vi "detect.vi"(0 "LS1":bool, 1 "Start":bool, 5 "LS2":bool, 7 "LS3":bool, 9 "LS4":bool, 11 "LS5":bool, 12 "Stop":bool) -> (6 "輸出":T1)   [LabVIEW 2014]
uses:
  state_D.ctl
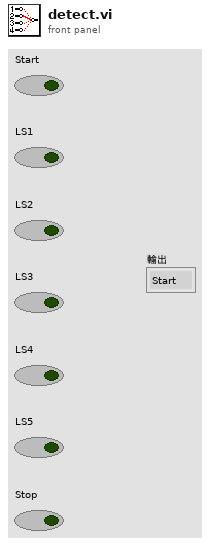
[diagram p1: front panel]
types:
  T1 = typedef "state_D.ctl" = enum16{"Start", "LS1", "LS2", "LS3", "LS4", "LS5", "Stop"}
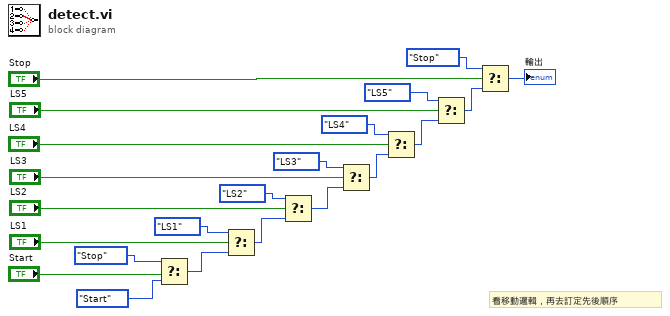
[diagram p0: block diagram]
diagram:
  # "看移動邏輯，再去訂定先後順序"
  n1 = Select(t=state_D."Stop", s="Start", f=state_D."Start") -> (s? t:f=w21:T1)
  n2 = Select(t=state_D."LS1", s="LS1", f=w21) -> (s? t:f=w20:T1)
  n3 = Select(t=state_D."LS2", s="LS2", f=w20) -> (s? t:f=w19:T1)
  n4 = Select(t=state_D."LS3", s="LS3", f=w19) -> (s? t:f=w14:T1)
  n5 = Select(t=state_D."LS4", s="LS4", f=w14) -> (s? t:f=w12:T1)
  n6 = Select(t=state_D."LS5", s="LS5", f=w12) -> (s? t:f=w10:T1)
  n7 = Select(t=state_D."Stop", s="Stop", f=w10) -> (s? t:f=→"輸出":T1)
